vi "Response String.vi"(8 "error in (no error)":errorcluster, 11 "Response in":refnum<class "Response.lvclass">) -> (0 "error out":errorcluster, 2 "Response String":string, 3 "Response out":refnum<class "Response.lvclass">)   [LabVIEW 2020, in "HTTP Utils.lvlib" / "Response.lvclass"]
uses:
  Response.lvclass
  Response.lvclass/Response.ctl
  Cookie/Cookie.lvclass
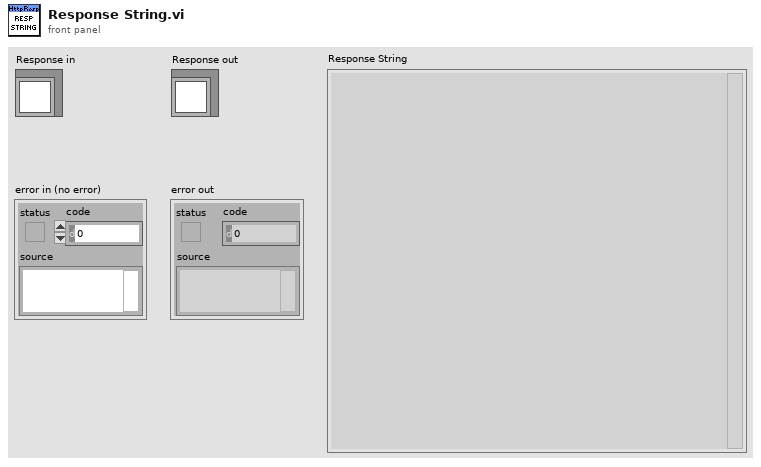
[diagram p1: front panel]
types:
  T1 = typedef "HTTP Utils.lvlib/Cookie Map.ctl" = map{string, refnum<class "Cookie.lvclass">}
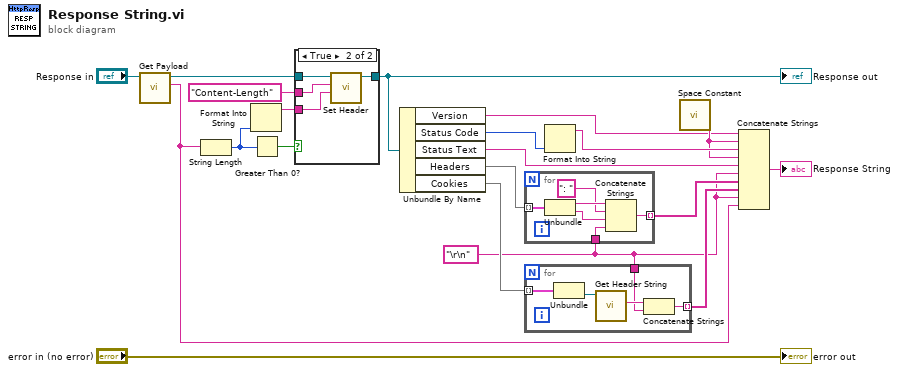
[diagram p0: block diagram]
diagram:
  w1 = "\r\n" ("string")
  n1 = call-dynamic "Get Payload.vi"("Response in"="Response in") -> ("Payload"=w3:string, "Response out"=w5:refnum<class "Response.lvclass">)  [unwired: 8 in, 1 out]
  n2 = String Length(string=w3) -> (length=w8:i32)
  n3 = Format Into String(w8) -> (resulting string=w19:string)  [unwired: 3 in, 1 out]
  n4 = Greater Than 0?(x=w8) -> (x > 0?=w7:bool)
  n5 = case shown="True" w7 {
    tunnel: w5 -> [w21 w25]
    tunnel: w19 -> [_ w24]
    tunnel: "Content-Length" ("Header") -> [_ w23]
    tunnel: [w21 w22] -> w9
    frame False {
    }
    frame True {
      n6 = call "Set Header.vi"("Value"=w24, "Header"=w23, "Response in"=w25) -> ("Response out"=w22:refnum<class "Response.lvclass">)  [unwired: 6 in, 2 out]
    }
  }
  "Response out" <- w9
  n7 = Unbundle By Name(w9) -> ("Version"=w11:string, "Status Code"=w14:u16, "Status Text"=w15:string, "Headers"=w17:map{string, string}, "Cookies"=w4:T1)
  n8 = for {
    tunnel: w17 -> [w31] mode=indexing
    tunnel: [w27] -> w16 mode=indexing
    tunnel: w1 -> [w26]
    n9 = Unbundle(w31) -> (w30:string, w28:string)
    n10 = Concatenate Strings(w30, ": " ("string"), w28, w26) -> (w27:string)
  }
  n11 = for {
    tunnel: w4 -> [w36] mode=indexing
    tunnel: [w35] -> w2 mode=indexing
    tunnel: w1 -> [w32]
    n12 = Unbundle(w36) -> ("Cookie"=w34:refnum<class "Cookie.lvclass">)  [unwired: 1 out]
    n13 = call "Get Header String.vi"("Cookie in"=w34) -> ("Header String"=w33:string)  [unwired: 8 in, 2 out]
    n14 = Concatenate Strings(w33, w32) -> (w35:string)
  }
  n15 = Format Into String(w14) -> (resulting string=w13:string)  [unwired: 3 in, 1 out]
  n16 = call <vilib>:"Space Constant.vi"() -> ("String"=w12:string)
  n17 = Concatenate Strings(w11, w12, w13, w12, w15, w1, w16, w2, w1, w3) -> (→"Response String":string)
  "error out" <- "error in (no error)"
